vi "aggregator - iii - real.vi"(5 "requested averaging interval":i32=10, 6 "first time":bool, 7 "requested size":i32=20, 8 "check for gtr than zero?":bool=TRUE, 11 "number":dbl) -> (0 "interpolated average":dbl, 1 "mean array":dbl[](array[numeric]), 2 "interp array":dbl[](array[numeric]), 3 "Array":dbl[](array[numeric]), 4 "slope":dbl)   [LabVIEW 2014]
panel:
  out "actual number of elements":i32
  out "mean":dbl
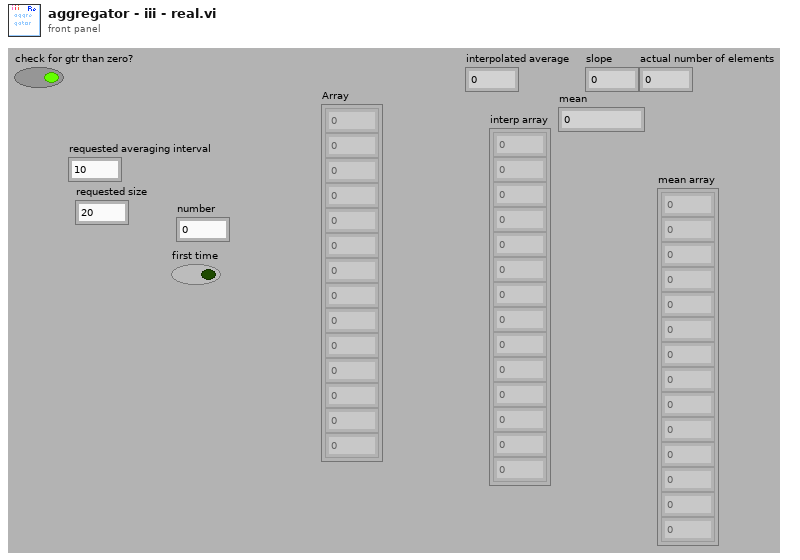
[diagram p1: front panel]
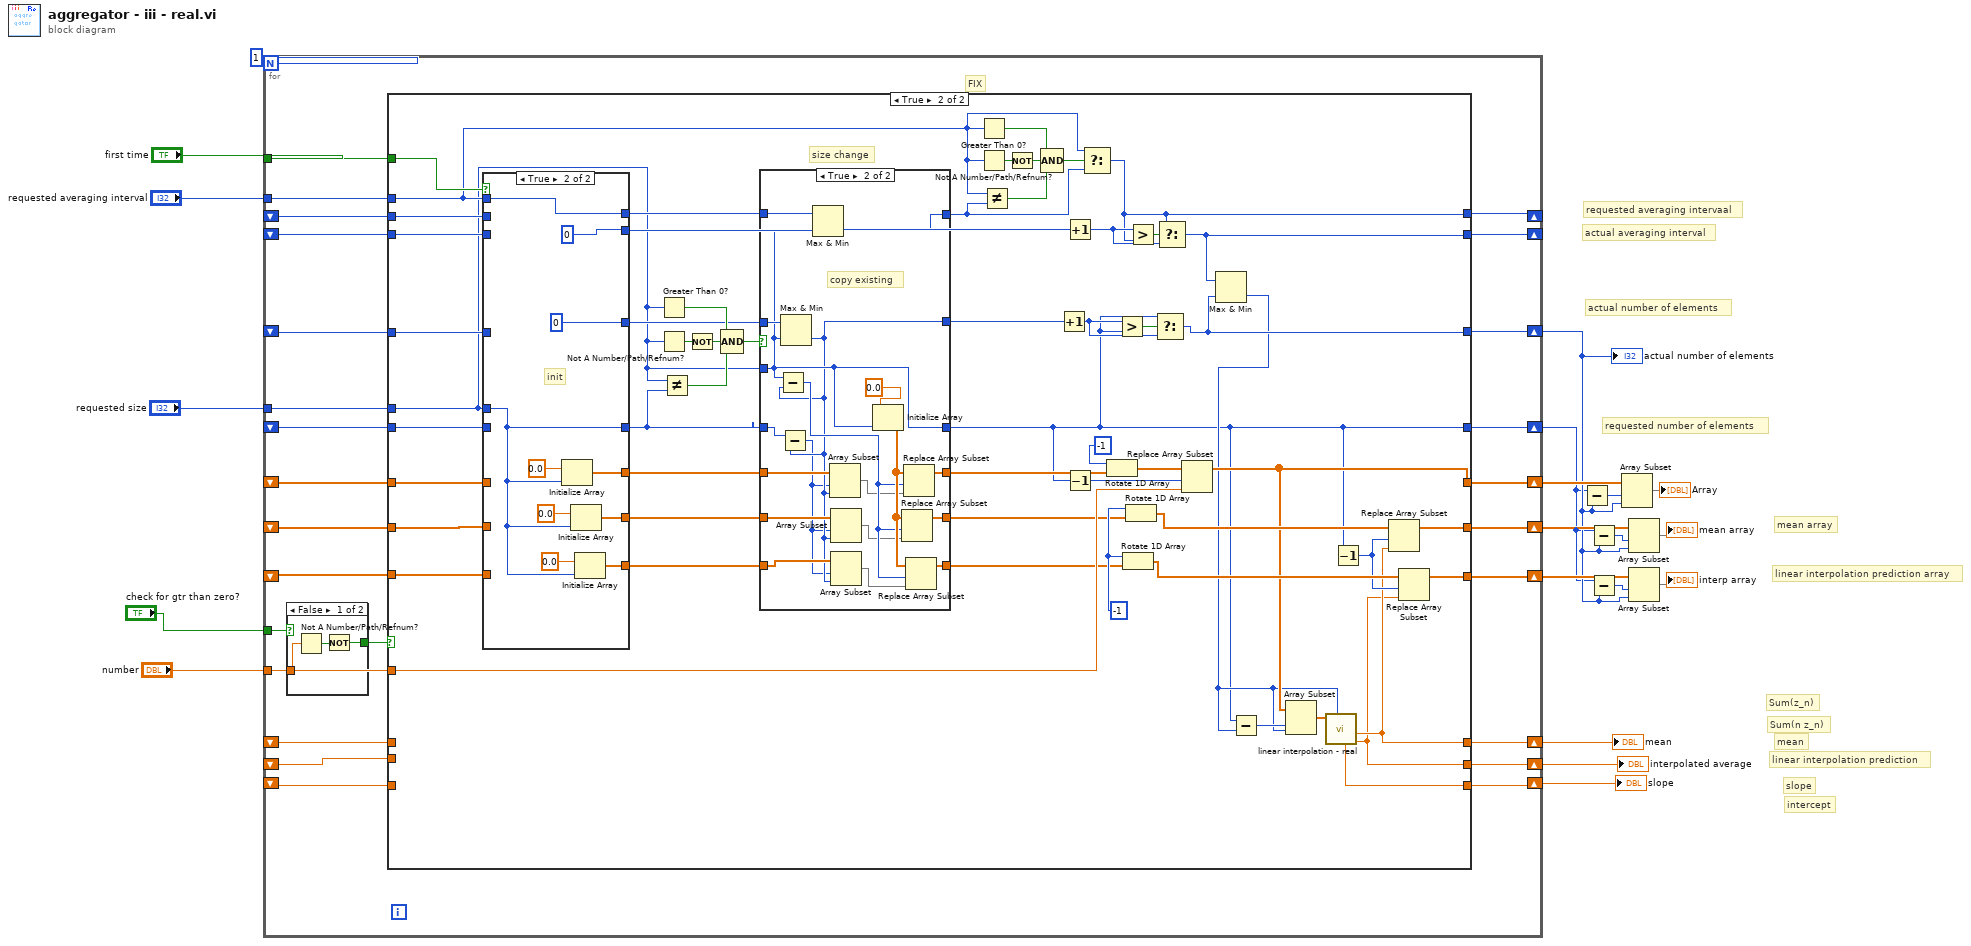
[diagram p0: block diagram]
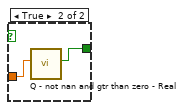
[diagram p2: hidden frame]
diagram:
  # "actual averaging interval"
  # "requested averaging intervaal"
  # "linear interpolation prediction"
  # "mean"
  # "intercept"
  # "slope"
  # "linear interpolation prediction array"
  # "mean array"
  # "Sum(n z_n)"
  # "Sum(z_n)"
  # "requested number of elements"
  # "actual number of elements"
  n1 = for {
    N: 1 -> [_]
    tunnel: "first time" -> [w36]
    shift-right: [w28] -> w6
    shift-left: _ -> [w46]
    tunnel: "requested size" -> [w32]
    tunnel: "number" -> [w26]
    shift-right: [w37] -> w16
    shift-left: _ -> [w45]
    shift-right: [w31] -> w5
    shift-left: _ -> [w44]
    shift-right: [w41] -> w10
    shift-left: _ -> [w43]
    shift-right: [w40] -> w7
    shift-left: _ -> [w42]
    shift-right: [w33] -> w3
    shift-left: _ -> [w23]
    shift-right: [w35] -> w2
    shift-left: _ -> [w25]
    shift-right: [w34] -> w4
    shift-left: _ -> [w24]
    shift-right: [w27] -> _
    shift-left: _ -> [w39]
    shift-right: [w29] -> _
    shift-left: _ -> [w38]
    tunnel: "requested averaging interval" -> [w30]
    tunnel: "check for gtr than zero?" -> [w21]
    # "FIX"
    n2 = case shown="False" w21 {
      tunnel: w26 -> [w49 w51]
      tunnel: [w47 w50] -> w22
      frame False {
        n3 = Not A Number/Path/Refnum?(number/path/refnum=w49) -> (NaN/Path/Refnum?=w48:bool)
        n4 = Not(x=w48) -> (.not. x?=w47:bool)
      }
      frame True {
        n5 = call "Q - not nan and gtr than zero - Real.vi"("Numeric"=w51) -> ("Boolean"=w50:bool)  [unwired: 9 in, 1 out]
      }
    }
    n6 = case shown="True" w22 {
      tunnel: w46 -> [w59 w118]
      tunnel: w45 -> [w57 w115]
      tunnel: w26 -> [_ w113]
      tunnel: w44 -> [w58 w110]
      tunnel: w43 -> [w56 w109]
      tunnel: w42 -> [w52 w108]
      tunnel: [w56 w103] -> w41
      tunnel: [w52 w102] -> w40
      tunnel: w39 -> [w60 w98]
      tunnel: w38 -> [w61 w97]
      tunnel: [w57 w96] -> w37
      tunnel: w36 -> [_ w94]
      tunnel: [w55 w92] -> w35
      tunnel: [w54 w91] -> w34
      tunnel: [w53 w90] -> w33
      tunnel: w32 -> [_ w71]
      tunnel: [w58 w63] -> w31
      tunnel: w30 -> [_ w80]
      tunnel: [w61 w79] -> w29
      tunnel: [w59 w78] -> w28
      tunnel: [w60 w77] -> w27
      tunnel: w25 -> [w55 _]
      tunnel: w24 -> [w54 _]
      tunnel: w23 -> [w53 _]
      frame False {
      }
      frame True {
        w105 = -1 ("n")
        # "size change"
        n7 = case shown="True" w94 {
          tunnel: w118 -> [w149 _]
          tunnel: [w149 0] -> w73
          tunnel: w115 -> [w146 _]
          tunnel: w71 -> [_ w151]
          tunnel: w110 -> [w147 _]
          tunnel: w109 -> [w145 _]
          tunnel: w108 -> [w144 _]
          tunnel: [w146 w154] -> w69
          tunnel: [w145 w153] -> w68
          tunnel: [w144 w152] -> w67
          tunnel: [w150 0] -> w100
          tunnel: w98 -> [w150 _]
          tunnel: w80 -> [_ w155]
          tunnel: w97 -> [w148 _]
          tunnel: [w148 w155] -> w74
          tunnel: [w147 w151] -> w70
          frame False {
          }
          frame True {
            # "init"
            n8 = Initialize Array(0.0, w151) -> (w154:dbl[])
            n9 = Initialize Array(0.0, w151) -> (w153:dbl[])
            n10 = Initialize Array(0.0, w151) -> (w152:dbl[])
          }
        }
        n11 = Greater Than 0?(x=w71) -> (x > 0?=w88:bool)
        n12 = Not A Number/Path/Refnum?(number/path/refnum=w71) -> (NaN/Path/Refnum?=w89:bool)
        n13 = Not Equal?(x=w71, y=w70) -> (x != y?=w86:bool)
        n14 = Not(x=w89) -> (.not. x?=w87:bool)
        n15 = Compound Arithmetic op=AND(w88, w87, w86) -> (w72:bool)
        n16 = case shown="True" w72 {
          tunnel: [w124 w126] -> w62
          tunnel: w73 -> [w124 w142]
          tunnel: [w123 w134] -> w63
          tunnel: w70 -> [w123 w127]
          tunnel: [w122 w141] -> w64
          tunnel: w69 -> [w122 w133]
          tunnel: w71 -> [_ w134]
          tunnel: w67 -> [w120 w131]
          tunnel: w68 -> [w121 w129]
          tunnel: [w121 w140] -> w65
          tunnel: [w120 w139] -> w66
          tunnel: w74 -> [w119 w136]
          tunnel: [w119 w135] -> w75
          frame False {
          }
          frame True {
            # "copy existing"
            n17 = Max & Min(x=w142, y=w134) -> (min(x,y)=w126:i32)  [unwired: 1 out]
            n18 = Subtract(x=w134, y=w126) -> (x-y=w137:i32)
            n19 = Subtract(x=w127, y=w126) -> (x-y=w125:i32)
            n20 = Max & Min(x=w136, y=w134) -> (min(x,y)=w135:i32)  [unwired: 1 out]
            n21 = Array Subset(array=w133, index=w125, length=w126) -> (w132:dbl[])
            n22 = Array Subset(array=w129, index=w125, length=w126) -> (w128:dbl[])
            n23 = Array Subset(array=w131, index=w125, length=w126) -> (w130:dbl[])
            n24 = Initialize Array(0.0, w134) -> (w138:dbl[])
            n25 = Replace Array Subset(array=w138, new element=w128, index=w137) -> (w140:dbl[])
            n26 = Replace Array Subset(array=w138, new element=w132, index=w137) -> (w141:dbl[])
            n27 = Replace Array Subset(array=w138, new element=w130, index=w137) -> (w139:dbl[])
          }
        }
        n28 = Greater Than 0?(x=w80) -> (x > 0?=w84:bool)
        n29 = Not A Number/Path/Refnum?(number/path/refnum=w80) -> (NaN/Path/Refnum?=w85:bool)
        n30 = Not Equal?(x=w80, y=w75) -> (x != y?=w82:bool)
        n31 = Not(x=w85) -> (.not. x?=w83:bool)
        n32 = Compound Arithmetic op=AND(w84, w83, w82) -> (w81:bool)
        n33 = Increment(x=w62) -> (x+1=w116:i32)
        n34 = Increment(x=w100) -> (x+1=w99:i32)
        n35 = Decrement(x=w63) -> (x-1=w112:i32)
        n36 = Select(t=w80, s=w81, f=w75) -> (s? t:f=w79:i32)
        n37 = Rotate 1D Array(1:w64, 2:-1 ("n")) -> (0:w111:dbl[])
        n38 = Greater?(x=w116, y=w63) -> (0:w117:bool)
        n39 = Rotate 1D Array(1:w66, 2:w105) -> (0:w106:dbl[])
        n40 = Rotate 1D Array(1:w65, 2:w105) -> (0:w107:dbl[])
        n41 = Greater?(x=w99, y=w79) -> (0:w101:bool)
        n42 = Select(t=w63, s=w117, f=w116) -> (s? t:f=w78:i32)
        n43 = Select(t=w79, s=w101, f=w99) -> (s? t:f=w77:i32)
        n44 = Replace Array Subset(array=w111, new element=w113, index=w112) -> (w96:dbl[])
        n45 = Max & Min(x=w77, y=w78) -> (min(x,y)=w76:i32)  [unwired: 1 out]
        n46 = Subtract(x=w63, y=w76) -> (x-y=w95:i32)
        n47 = Array Subset(array=w96, index=w95, length=w76) -> (w93:dbl[])
        n48 = call "linear interpolation - real.vi"("n"=w76, "Array"=w93) -> ("interpolated average"=w91:dbl, "mean"=w92:dbl, "slope"=w90:dbl)  [unwired: 4 in, 3 out]
        n49 = Decrement(x=w63) -> (x-1=w104:i32)
        n50 = Replace Array Subset(array=w107, new element=w92, index=w104) -> (w103:dbl[])
        n51 = Replace Array Subset(array=w106, new element=w91, index=w104) -> (w102:dbl[])
      }
    }
  }
  "interpolated average" <- w4
  "slope" <- w3
  "mean" <- w2
  "actual number of elements" <- w6
  n52 = Subtract(x=w5, y=w6) -> (x-y=w14:i32)
  n53 = Subtract(x=w5, y=w6) -> (x-y=w11:i32)
  n54 = Subtract(x=w5, y=w6) -> (x-y=w8:i32)
  n55 = Array Subset(array=w16, index=w14, length=w6) -> (→"Array":dbl[])
  n56 = Array Subset(array=w10, index=w11, length=w6) -> (→"mean array":dbl[])
  n57 = Array Subset(array=w7, index=w8, length=w6) -> (→"interp array":dbl[])
